vi "STOP Message Create.vi"(8 "error in (no error)":errorcluster, 11 "STOP in":refnum<class "STOP.lvclass">) -> (0 "error out":errorcluster, 3 "STOP out":refnum<class "STOP.lvclass">)   [LabVIEW 2018, in "STOP.lvclass"]
uses:
  STOP.lvclass
  C:/Users/aaron.jencks/Documents/GitHub/emerson_seed_object_detection/LabVIEW/Projects/Paul's Video Viewer/Classes/Message/Message.lvclass
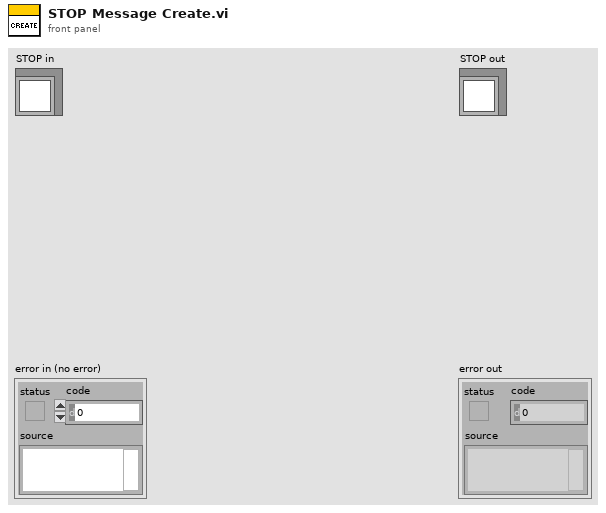
[diagram p1: front panel]
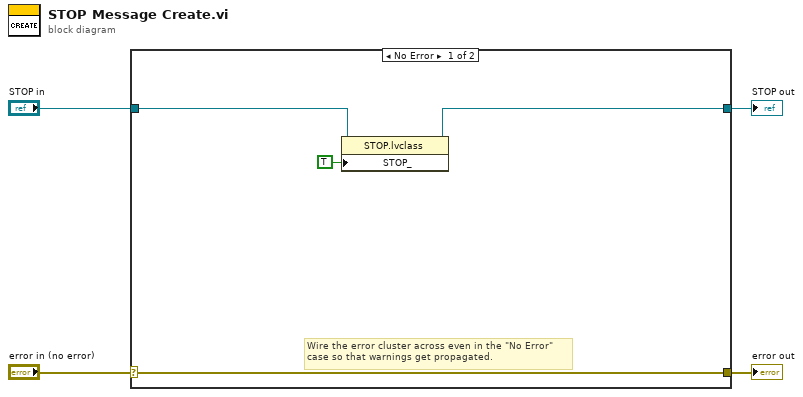
[diagram p0: block diagram]
diagram:
  n1 = case shown="No Error" "error in (no error)" {
    selector: "error in (no error)" -> [w8 w10]
    tunnel: [w8 w10] -> w3
    tunnel: [w6 w9] -> w1
    tunnel: "STOP in" -> [w7 w9]
    frame No Error {
      # "Wire the error cluster across even in the \"No Error\"\ncase so that warnings get propagated."
      n2 = property class="STOP.lvclass"(reference=w7, "STOP_"=TRUE) -> (reference out=w6:refnum<class "STOP.lvclass">)  [unwired: 1 in, 1 out]
    }
    frame Error {
    }
  }
  "error out" <- w3
  "STOP out" <- w1
